vi "Begin.vi"(8 "error in":errorcluster) -> (0 "error out":errorcluster)   [LabVIEW 2019]
doc: "Called before other user functions, this VI is expected to open initial I/O refnums, load in file data, and do all program initialization. Notice that the <B>error out</B> terminal is simply used for data flow. Wiring it to other structures or subVIs ensures that this VI runs first."
uses:
  <vilib>/Rock Robotics/WPI/SafetyOutput/WPI_SafetyOutputConfigMenu.ctl
  <vilib>/Rock Robotics/WPI/DriverStation/WPI_DriverStationRobotMode2.ctl
  <vilib>/Rock Robotics/WPI/Joystick/WPI_JoystickDeviceEnum.ctl
  Robot Global Data.vi
  <vilib>/Rock Robotics/Network Tables/NT Write String Array.vi
  <vilib>/Rock Robotics/WPI/ThirdParty/Phoenix-LabVIEW/Motor Controller/Controls/CTRE_Phoenix_MotorControl_ControlMode.ctl
  <vilib>/Utility/file.llb/Read Delimited Spreadsheet (DBL).vi
  <vilib>/Rock Robotics/WPI/ThirdParty/Phoenix-LabVIEW/Motor Controller/Controls/CTRE_Phoenix_MotorControl_MotionProfileTrajectoryPoint.ctl
  <vilib>/Rock Robotics/WPI/ThirdParty/Phoenix-LabVIEW/Motor Controller/Closed Loop/Motion Profile/CTRE_Phoenix_MotorControl_BufferedTrajectoryPointStream_WriteAll.vi
  <vilib>/Rock Robotics/WPI/ThirdParty/Phoenix-LabVIEW/Motor Controller/Controls/CTRE_Phoenix_MotorControl_FeedbackDevice.ctl
  <vilib>/Rock Robotics/WPI/RobotDrive/WPI_RobotDriveOpen2MotorWithExistingMotors.vi
panel:
  in  "PID":T1
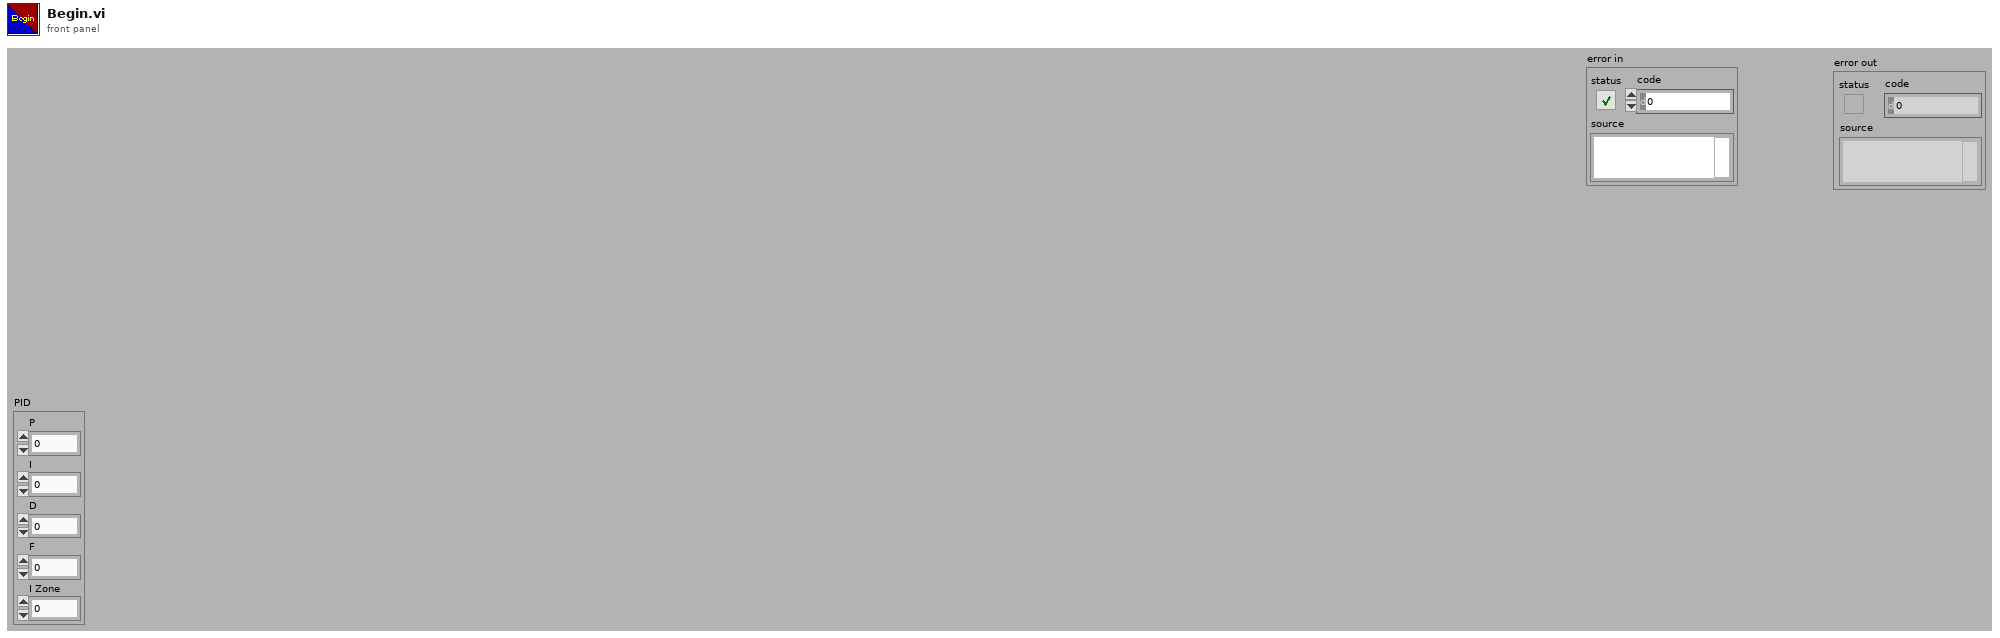
[diagram p1: front panel]
types:
  T1 = cluster{"P":dbl, "I":dbl, "D":dbl, "F":dbl, "I Zone":dbl}
  T2 = enum16{"FollowerType_PercentOutput", "FollowerType_AuxOutput1"}
  T3 = typedef "CTRE_Phoenix_MotorControl_FeedbackDevice.ctl" = i8
  T4 = typedef "CTRE_Phoenix_MotorControl_ControlMode.ctl" = u16
  T5 = typedef "WPI_JoystickDeviceEnum.ctl" = enum16{"USB 0", "USB 1", "USB 2", "USB 3", "USB 4", "USB 5"}
  T6 = typedef "WPI_SafetyOutputConfigMenu.ctl" = enum16{"Enable", "Disable"}
  T7 = typedef "WPI_DriverStationRobotMode2.ctl" = enum16{"Autonomous Disabled", "Autonomous Enabled", "Teleop Disabled", "Teleop Enabled", "Disconnected", "Finish", "Test Disabled", "Test Enabled", "Emergency Stopped"}
  T8 = typedef "WPI_MotorControlDeviceRef.ctl" = cluster{"DeviceStatus":errorcluster, "Type":T9, "PWM":cluster{"PWM Channel":T10, "DeadBand":T11}, "CAN":cluster{"Device Number":u8, "SetOutput VI Ref":variant, "GetOutput VI Ref":variant, "Enable VI Ref":variant, "Disable VI Ref":variant, "Data":variant}, "Invert":bool, "DIO PWM":cluster{"PWM \"Enable\" Channel":T10, "DIOChannel":T12, "PWM Rate":dbl}}
  T9 = typedef "WPI_MotorControlType.ctl" = enum16{"PWM", "CAN", "DIO PWM"}
  T10 = typedef "FPGA_DIOPWMChannel.ctl" = enum8{"PWM 0", "PWM 1", "PWM 2", "PWM 3", "PWM 4", "PWM 5", "PWM 6", "PWM 7", "PWM 8", "PWM 9", "PWM MXP 0", "PWM MXP 1", "PWM MXP 2", "PWM MXP 3", "PWM MXP 4", "PWM MXP 5", "PWM MXP 6", "PWM MXP 7", "PWM MXP 8", "PWM MXP 9", "Invalid"}
  T11 = typedef "WPI_PWMDeadband.ctl" = cluster{"Name":string, "maxPositivePwm":i32, "minPositivePwm":i32, "centerPwm":i32, "maxNegativePwm":i32, "minNegativePwm":i32, "angularRange":u16}
  T12 = typedef "FPGA_DIOChannel.ctl" = enum8{"DIO 0", "DIO 1", "DIO 2", "DIO 3", "DIO 4", "DIO 5", "DIO 6", "DIO 7", "DIO 8", "DIO 9", "DIO MXP 0", "DIO MXP 1", "DIO MXP 2", "DIO MXP 3", "DIO MXP 4", "DIO MXP 5", "DIO MXP 6", "DIO MXP 7", "DIO MXP 8", "DIO MXP 9", "DIO MXP 10", "DIO MXP 11", "DIO MXP 12", "DIO MXP 13", "DIO MXP 14", "DIO MXP 15", "SPI Port CS1", "SPI Port CS2", "SPI Port CS3", "SPI Port MISO", "SPI Port MOSI", "Invalid"}
  T13 = typedef "WPI_RobotDriveDevRef.ctl" = cluster{"DevStatus":errorcluster, "Motors[]":T8[], "Square Inputs":bool, "Max Output":dbl}
  T14 = typedef "WPI_JoystickDevRef.ctl" = cluster{"Device":T5}
  T15 = typedef "CTRE_Phoenix_MotorControl_MotionProfileTrajectoryPoint.ctl" = cluster{"Position":dbl, "Velocity":dbl, "Arbitrary Feed Forward":dbl, "Auxiliary Position":dbl, "Auxiliary Velocity":dbl, "Auxiliary Arbitrary Feed Forward":dbl, "Profile Slot Select":i32, "Auxiliary Profile Slot Select":i32, "isLastPoint?":bool, "Zero Position?":bool, "durationMs":u32, "Use Aux PID?":bool}
  T16 = typedef "CTRE_Phoenix_MotorControl_BufferedTrajectoryPointStream_DeviceRef.ctl" = cluster{"Handle":u64, "Library Path":path}
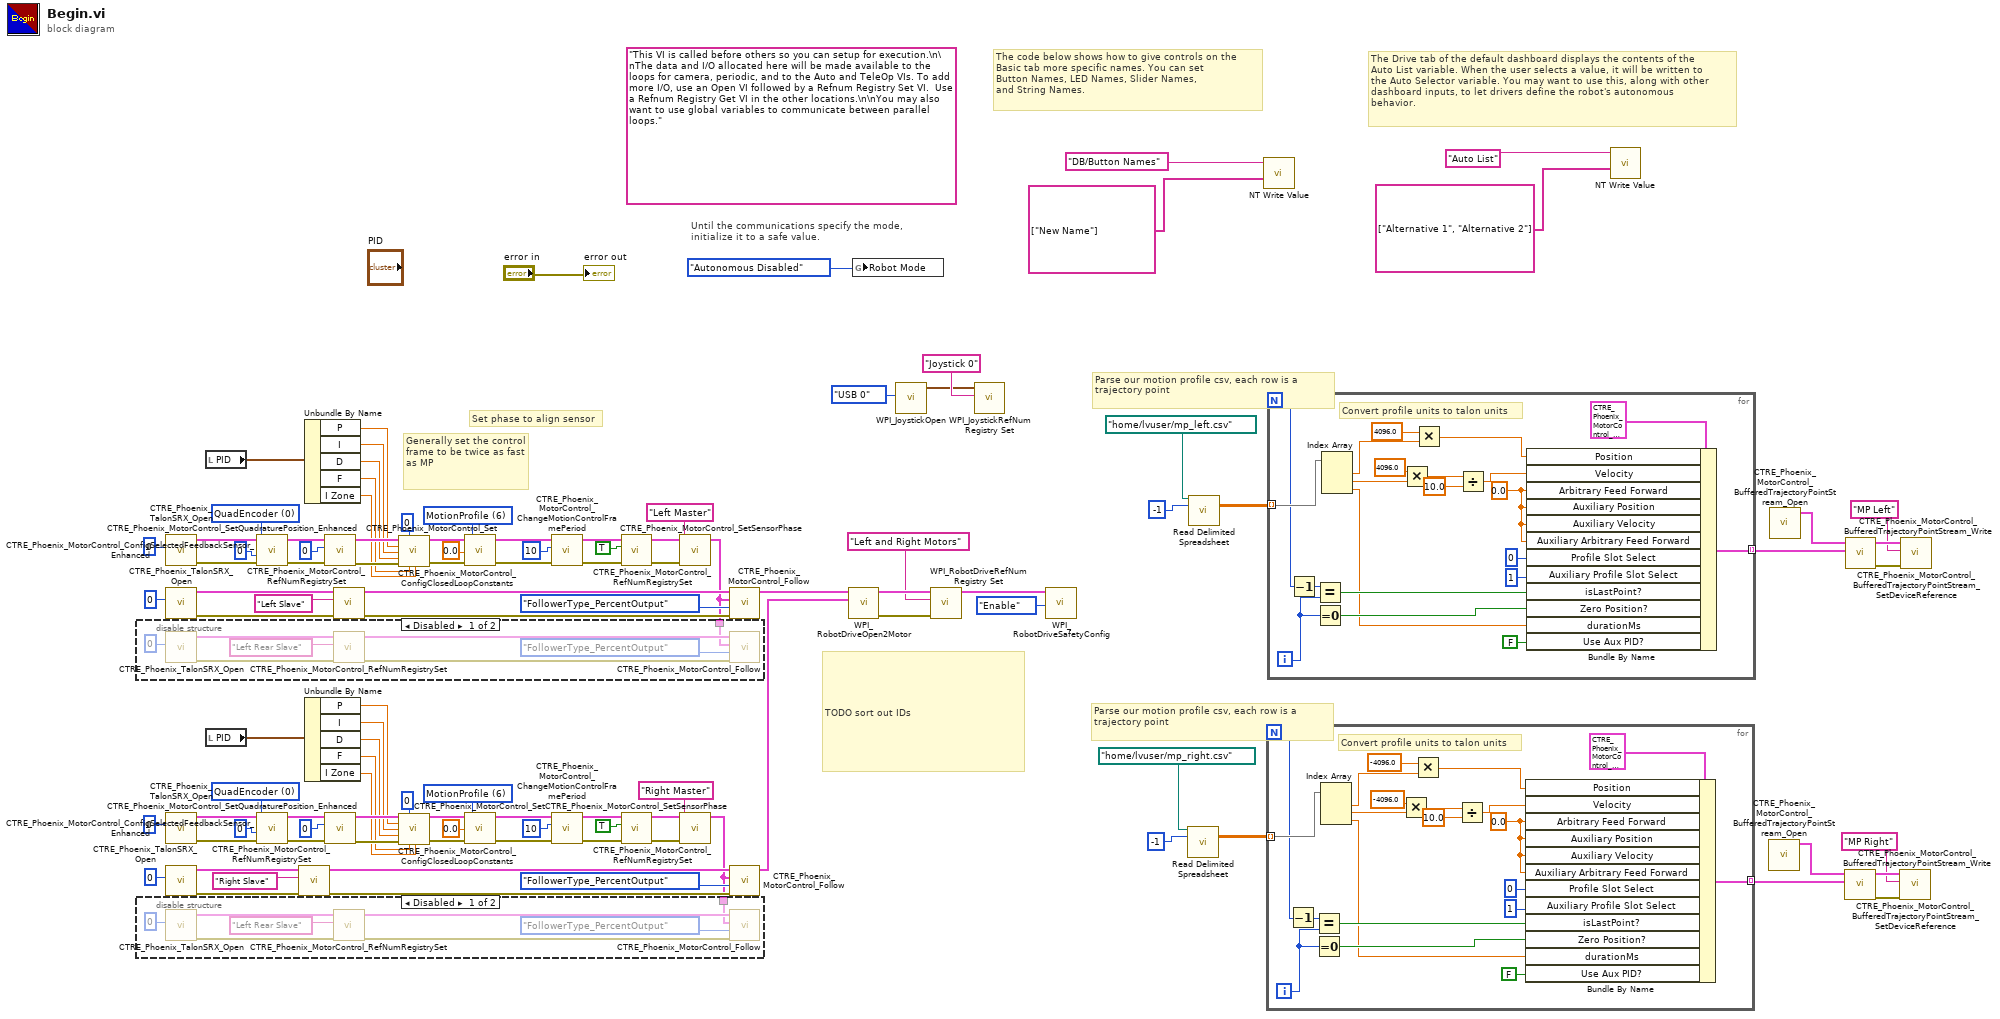
[diagram p0: block diagram]
diagram:
  w40 = T3 0 items=["QuadEncoder"=0, "Analog"=2, "Tachometer"=4, "Pulse Width Encoded Position"=8, "Sensor Sum (S0 + S1)"=9, "Sensor Difference (D0 - D1)"=10, "Remote Source 0"=11, "Remote Source 1"=12, "Software Emulated"=15] ("Feedback Device")
  w48 = T4 6 items=["PercentOutput"=0, "Position"=1, "Velocity"=2, "Current"=3, "Follower"=5, "MotionProfile"=6, "MotionMagic"=7, "MotionMagicArc"=8, "MotionProfileArc"=10, "Disabled"=15] ("Control Mode")
  w77 = T3 0 items=["QuadEncoder"=0, "Analog"=2, "Tachometer"=4, "Pulse Width Encoded Position"=8, "Sensor Sum (S0 + S1)"=9, "Sensor Difference (D0 - D1)"=10, "Remote Source 0"=11, "Remote Source 1"=12, "Software Emulated"=15] ("Feedback Device")
  w93 = T4 6 items=["PercentOutput"=0, "Position"=1, "Velocity"=2, "Current"=3, "Follower"=5, "MotionProfile"=6, "MotionMagic"=7, "MotionMagicArc"=8, "MotionProfileArc"=10, "Disabled"=15] ("Control Mode")
  (unwired) "This VI is called before others so you can setup for execution.\n\nThe data and I/O allocated here will be made available to the loops for camera, periodic, and to the Auto and TeleOp VIs. To add more I/O, use an Open VI followed by a Refnum Registry Set VI.  Use a Refnum Registry Get VI in the other locations.\n\nYou may also want to use global variables to communicate between parallel loops."
  # "Parse our motion profile csv, each row is a trajectory point"
  # "TODO sort out IDs"
  # "Set phase to align sensor"
  # "Generally set the control frame to be twice as fast as MP"
  # "Parse our motion profile csv, each row is a trajectory point"
  # "The Drive tab of the default dashboard displays the contents of the\nAuto List variable. When the user selects a value, it will be written to\nthe Auto Selector variable. You may want to use this, along with other\ndashboard inputs, to let drivers define the robot's autonomous\nbehavior."
  # "The code below shows how to give controls on the\nBasic tab more specific names. You can set\nButton Names, LED Names, Slider Names,\nand String Names."
  # "Until the communications specify the mode,\ninitialize it to a safe value."
  n1 = call <vilib>:"CTRE_Phoenix_TalonSRX_Open.vi"("Device Number"=u8 0) -> ("error out"=w79:errorcluster, "CAN Talon SRX Ref"=w78:T8)  [unwired: 9 in]
  n2 = call <vilib>:"CTRE_Phoenix_TalonSRX_Open.vi"("Device Number"=u8 0) -> ("error out"=w54:errorcluster, "CAN Talon SRX Ref"=w55:T8)  [unwired: 9 in]
  n3 = call <vilib>:"CTRE_Phoenix_TalonSRX_Open.vi"("Device Number"=u8 0) -> ("error out"=w42:errorcluster, "CAN Talon SRX Ref"=w41:T8)  [unwired: 9 in]
  n4 = call <vilib>:"CTRE_Phoenix_TalonSRX_Open.vi"("Device Number"=u8 0) -> ("error out"=w17:errorcluster, "CAN Talon SRX Ref"=w18:T8)  [unwired: 9 in]
  n5 = local read "PID"() -> (w60:T1)
  n6 = local read "PID"() -> (w23:T1)
  n7 = call <vilib>:"CTRE_Phoenix_MotorControl_ConfigSelectedFeedbackSensor_Enhanced.vi"("error in (no error)"=w79, "pidLoopIdx"=0, "Feedback Device"=w77, "PhoenixMotorControlDevRef"=w78) -> ("error out"=w74:errorcluster, "PhoenixMotorControlDevRef"=w75:T8)  [unwired: 6 in]
  n8 = call <vilib>:"CTRE_Phoenix_MotorControl_ConfigSelectedFeedbackSensor_Enhanced.vi"("error in (no error)"=w42, "pidLoopIdx"=0, "Feedback Device"=w40, "PhoenixMotorControlDevRef"=w41) -> ("error out"=w37:errorcluster, "PhoenixMotorControlDevRef"=w38:T8)  [unwired: 6 in]
  n9 = call <vilib>:"CTRE_Phoenix_MotorControl_RefNumRegistrySet.vi"("error in (no error)"=w17, "refnum name"="Right Slave", "PhoenixMotorControlDevRef"=w18) -> ("error out"=w13:errorcluster, "PhoenixMotorControlDevRef"=w15:T8)  [unwired: 7 in]
  n10 = Unbundle By Name(w60) -> ("P"=w70:dbl, "I"=w69:dbl, "D"=w68:dbl, "F"=w67:dbl, "I Zone"=w66:dbl)
  n11 = Unbundle By Name(w23) -> ("P"=w33:dbl, "I"=w32:dbl, "D"=w31:dbl, "F"=w30:dbl, "I Zone"=w29:dbl)
  n12 = call <vilib>:"CTRE_Phoenix_MotorControl_SetQuadraturePosition_Enhanced.vi"("error in (no error)"=w74, "New Position"=0, "PhoenixMotorControlDevRef"=w75) -> ("error out"=w71:errorcluster, "PhoenixMotorControlDevRef"=w72:T8)  [unwired: 7 in]
  n13 = call <vilib>:"CTRE_Phoenix_MotorControl_SetQuadraturePosition_Enhanced.vi"("error in (no error)"=w37, "New Position"=0, "PhoenixMotorControlDevRef"=w38) -> ("error out"=w34:errorcluster, "PhoenixMotorControlDevRef"=w35:T8)  [unwired: 7 in]
  n14 = call <vilib>:"CTRE_Phoenix_MotorControl_RefNumRegistrySet.vi"("error in (no error)"=w54, "refnum name"="Left Slave", "PhoenixMotorControlDevRef"=w55) -> ("error out"=w50:errorcluster, "PhoenixMotorControlDevRef"=w52:T8)  [unwired: 7 in]
  n15 = call <vilib>:"CTRE_Phoenix_MotorControl_ConfigClosedLoopConstants.vi"("PhoenixMotorControlDevRef"=w72, "slotIdx"=0, "P"=w70, "I"=w69, "D"=w68, "error in (no error)"=w71, "F"=w67, "I Zone"=w66) -> ("PhoenixMotorControlDevRef"=w64:T8, "error out"=w63:errorcluster)  [unwired: 6 in]
  n16 = call <vilib>:"CTRE_Phoenix_MotorControl_ConfigClosedLoopConstants.vi"("PhoenixMotorControlDevRef"=w35, "slotIdx"=0, "P"=w33, "I"=w32, "D"=w31, "error in (no error)"=w34, "F"=w30, "I Zone"=w29) -> ("PhoenixMotorControlDevRef"=w27:T8, "error out"=w26:errorcluster)  [unwired: 6 in]
  n17 = call <vilib>:"CTRE_Phoenix_MotorControl_Set.vi"("error in (no error)"=w63, "Output"=0.0, "Control Mode"=w93, "PhoenixMotorControlDevRef"=w64) -> ("error out"=w62:errorcluster, "PhoenixMotorControlDevRef"=w82:T8)  [unwired: 6 in]
  n18 = call <vilib>:"CTRE_Phoenix_MotorControl_Set.vi"("error in (no error)"=w26, "Output"=0.0, "Control Mode"=w48, "PhoenixMotorControlDevRef"=w27) -> ("error out"=w25:errorcluster, "PhoenixMotorControlDevRef"=w45:T8)  [unwired: 6 in]
  n19 = call <vilib>:"CTRE_Phoenix_MotorControl_ChangeMotionControlFramePeriod.vi"("error in"=w62, "periodMs"=10, "PhoenixMotorControlDevRef"=w82) -> ("error out"=w61:errorcluster, "PhoenixMotorControlDevRef"=w80:T8)  [unwired: 7 in]
  n20 = call <vilib>:"CTRE_Phoenix_MotorControl_ChangeMotionControlFramePeriod.vi"("error in"=w25, "periodMs"=10, "PhoenixMotorControlDevRef"=w45) -> ("error out"=w24:errorcluster, "PhoenixMotorControlDevRef"=w43:T8)  [unwired: 7 in]
  n21 = call <vilib>:"CTRE_Phoenix_MotorControl_SetSensorPhase.vi"("error in (no error)"=w61, "PhaseSensor"=TRUE, "PhoenixMotorControlDevRef"=w80) -> ("error out"=w59:errorcluster, "PhoenixMotorControlDevRef"=w58:T8)  [unwired: 7 in]
  n22 = call <vilib>:"CTRE_Phoenix_MotorControl_SetSensorPhase.vi"("error in (no error)"=w24, "PhaseSensor"=TRUE, "PhoenixMotorControlDevRef"=w43) -> ("error out"=w22:errorcluster, "PhoenixMotorControlDevRef"=w21:T8)  [unwired: 7 in]
  n23 = call <vilib>:"CTRE_Phoenix_MotorControl_RefNumRegistrySet.vi"("error in (no error)"=w59, "refnum name"="Left Master", "PhoenixMotorControlDevRef"=w58) -> ("PhoenixMotorControlDevRef"=w2:T8)  [unwired: 7 in, 1 out]
  n24 = disable-structure shown="Disabled" {
    disable-tunnel: w2 -> [w109 _]
    frame Disabled {
      n25 = call <vilib>:"CTRE_Phoenix_TalonSRX_Open.vi"("Device Number"=u8 0) -> ("error out"=w114:errorcluster, "CAN Talon SRX Ref"=w115:T8)  [unwired: 9 in]
      n26 = call <vilib>:"CTRE_Phoenix_MotorControl_RefNumRegistrySet.vi"("error in (no error)"=w114, "refnum name"="Left Rear Slave", "PhoenixMotorControlDevRef"=w115) -> ("error out"=w110:errorcluster, "PhoenixMotorControlDevRef"=w112:T8)  [unwired: 7 in]
      n27 = call <vilib>:"CTRE_Phoenix_MotorControl_Follow.vi"("error in (no error)"=w110, "FollowerType"=T2."FollowerType_PercentOutput", "Master Controller to Follow"=w109, "PhoenixMotorControlDevRef"=w112) -> ()  [unwired: 6 in, 2 out]
    }
    frame Enabled {
    }
  }
  n28 = call <vilib>:"CTRE_Phoenix_MotorControl_RefNumRegistrySet.vi"("error in (no error)"=w22, "refnum name"="Right Master", "PhoenixMotorControlDevRef"=w21) -> ("PhoenixMotorControlDevRef"=w1:T8)  [unwired: 7 in, 1 out]
  n29 = disable-structure shown="Disabled" {
    disable-tunnel: w1 -> [w117 _]
    frame Disabled {
      n30 = call <vilib>:"CTRE_Phoenix_TalonSRX_Open.vi"("Device Number"=u8 0) -> ("error out"=w122:errorcluster, "CAN Talon SRX Ref"=w123:T8)  [unwired: 9 in]
      n31 = call <vilib>:"CTRE_Phoenix_MotorControl_RefNumRegistrySet.vi"("error in (no error)"=w122, "refnum name"="Left Rear Slave", "PhoenixMotorControlDevRef"=w123) -> ("error out"=w118:errorcluster, "PhoenixMotorControlDevRef"=w120:T8)  [unwired: 7 in]
      n32 = call <vilib>:"CTRE_Phoenix_MotorControl_Follow.vi"("error in (no error)"=w118, "FollowerType"=T2."FollowerType_PercentOutput", "Master Controller to Follow"=w117, "PhoenixMotorControlDevRef"=w120) -> ()  [unwired: 6 in, 2 out]
    }
    frame Enabled {
    }
  }
  n33 = call <vilib>:"CTRE_Phoenix_MotorControl_Follow.vi"("error in (no error)"=w50, "FollowerType"=T2."FollowerType_PercentOutput", "Master Controller to Follow"=w2, "PhoenixMotorControlDevRef"=w52) -> ("PhoenixMotorControlDevRef"=w12:T8)  [unwired: 6 in, 1 out]
  n34 = call <vilib>:"CTRE_Phoenix_MotorControl_Follow.vi"("error in (no error)"=w13, "FollowerType"=T2."FollowerType_PercentOutput", "Master Controller to Follow"=w1, "PhoenixMotorControlDevRef"=w15) -> ("PhoenixMotorControlDevRef"=w11:T8)  [unwired: 6 in, 1 out]
  n35 = call-poly <vilib>:"WPI_RobotDriveOpen2Motor.vi"("Right Motor Dev Ref"=w11, "Left Motor Dev Ref"=w12) -> ("error out"=w100:errorcluster, "RobotDriveDevRef"=w102:T13)  [unwired: 3 in, 5 out]
  n36 = global write "Robot Global Data.vi" "Robot Mode"(WPI_DriverStationRobotMode2."Autonomous Disabled" ("Robot Mode")) -> ()
  n37 = call <vilib>:"WPI_JoystickOpen.vi"("JoystickDevice"=WPI_JoystickDeviceEnum."USB 0") -> ("JoystickDevRef"=w96:T14)  [unwired: 10 in]
  n38 = call <vilib>:"WPI_RobotDriveRefNum Registry Set.vi"("error in (no error)"=w100, "refnum name"="Left and Right Motors", "RobotDriveDevRef"=w102) -> ("RobotDriveDevRef"=w99:T13)  [unwired: 1 in, 7 out]
  n39 = call <vilib>:"WPI_JoystickRefNum Registry Set.vi"("refnum name"="Joystick 0", "JoystickDevRef"=w96) -> ()  [unwired: 8 in, 2 out]
  n40 = call <vilib>:"WPI_RobotDriveSafetyConfig.vi"("mode"=WPI_SafetyOutputConfigMenu."Enable", "RobotDriveDevRef"=w99) -> ()  [unwired: 8 in, 2 out]
  n41 = call-poly <vilib>:"Read Delimited Spreadsheet.vi"("file path (dialog if empty)"=path "/home/lvuser/mp_right.csv" ("file path (use dialog)"), "number of rows (all:-1)"=-1) -> ("all rows"=w8:dbl[][])  [unwired: 8 in, 5 out]
  n42 = call-poly <vilib>:"Read Delimited Spreadsheet.vi"("file path (dialog if empty)"=path "/home/lvuser/mp_left.csv" ("file path (use dialog)"), "number of rows (all:-1)"=-1) -> ("all rows"=w89:dbl[][])  [unwired: 8 in, 5 out]
  n43 = call-poly <vilib>:"NT Write Value.vi"("String Array"=string[] ["New Name"], "Name"="DB/Button Names") -> ()  [unwired: 9 in, 1 out]
  n44 = for {
    N -> [w138]
    tunnel: w8 -> [w144] mode=indexing
    tunnel: [w134] -> w7 mode=indexing
    i -> [w137]
    w143 = 0.0 ("Arbitrary Feed Forward")
    # "Convert profile units to talon units"
    n45 = Decrement(x=w138) -> (x-1=w139:i32)
    n46 = Equal?(x=w139, y=w137) -> (x = y?=w140:bool)
    n47 = Equal To 0?(x=w137) -> (x = 0?=w136:bool)
    n48 = Index Array(array=w144) -> (element #1=w132:dbl, element #2=w126:dbl, element #3=w133:dbl)  [unwired: 3 in]
    n49 = Multiply(x=-4096.0, y=w126) -> (x*y=w128:dbl)
    n50 = Multiply(x=-4096.0, y=w132) -> (x*y=w130:dbl)
    n51 = Divide(x=w128, y=10.0) -> (x/y=w125:dbl)
    n52 = Bundle By Name(cluster=T15 {"Position"=0.0, "Velocity"=0.0, "Arbitrary Feed Forward"=0.0, "Auxiliary Position"=0.0, "Auxiliary Velocity"=0.0, "Auxiliary Arbitrary Feed Forward"=0.0, "Profile Slot Select"=0, "Auxiliary Profile Slot Select"=0, "isLastPoint?"=FALSE, "Zero Position?"=FALSE, "durationMs"=0, "Use Aux PID?"=FALSE} ("Trajectory Point"), "Position"=w130, "Velocity"=w125, "Arbitrary Feed Forward"=w143, "Auxiliary Position"=w143, "Auxiliary Velocity"=w143, "Auxiliary Arbitrary Feed Forward"=w143, "Profile Slot Select"=0, "Auxiliary Profile Slot Select"=1, "isLastPoint?"=w140, "Zero Position?"=w136, "durationMs"=w133, "Use Aux PID?"=FALSE) -> (w134:T15)
  }
  n53 = for {
    N -> [w159]
    tunnel: w89 -> [w165] mode=indexing
    tunnel: [w155] -> w88 mode=indexing
    i -> [w158]
    w164 = 0.0 ("Arbitrary Feed Forward")
    # "Convert profile units to talon units"
    n54 = Decrement(x=w159) -> (x-1=w160:i32)
    n55 = Equal?(x=w160, y=w158) -> (x = y?=w161:bool)
    n56 = Equal To 0?(x=w158) -> (x = 0?=w157:bool)
    n57 = Index Array(array=w165) -> (element #1=w153:dbl, element #2=w147:dbl, element #3=w154:dbl)  [unwired: 3 in]
    n58 = Multiply(x=4096.0, y=w147) -> (x*y=w149:dbl)
    n59 = Multiply(x=4096.0, y=w153) -> (x*y=w151:dbl)
    n60 = Divide(x=w149, y=10.0) -> (x/y=w146:dbl)
    n61 = Bundle By Name(cluster=T15 {"Position"=0.0, "Velocity"=0.0, "Arbitrary Feed Forward"=0.0, "Auxiliary Position"=0.0, "Auxiliary Velocity"=0.0, "Auxiliary Arbitrary Feed Forward"=0.0, "Profile Slot Select"=0, "Auxiliary Profile Slot Select"=0, "isLastPoint?"=FALSE, "Zero Position?"=FALSE, "durationMs"=0, "Use Aux PID?"=FALSE} ("Trajectory Point"), "Position"=w151, "Velocity"=w146, "Arbitrary Feed Forward"=w164, "Auxiliary Position"=w164, "Auxiliary Velocity"=w164, "Auxiliary Arbitrary Feed Forward"=w164, "Profile Slot Select"=0, "Auxiliary Profile Slot Select"=1, "isLastPoint?"=w161, "Zero Position?"=w157, "durationMs"=w154, "Use Aux PID?"=FALSE) -> (w155:T15)
  }
  n62 = call-poly <vilib>:"NT Write Value.vi"("String Array"=string[] ["Alternative 1", "Alternative 2"], "Name"="Auto List") -> ()  [unwired: 9 in, 1 out]
  n63 = call <vilib>:"CTRE_Phoenix_MotorControl_BufferedTrajectoryPointStream_Open.vi"() -> ("BufferedTrajectoryPointStream_DevRef"=w6:T16)  [unwired: 10 in, 1 out]
  n64 = call <vilib>:"CTRE_Phoenix_MotorControl_BufferedTrajectoryPointStream_Open.vi"() -> ("BufferedTrajectoryPointStream_DevRef"=w87:T16)  [unwired: 10 in, 1 out]
  n65 = call-poly <vilib>:"CTRE_Phoenix_MotorControl_BufferedTrajectoryPointStream_Write.vi"("Motion Profile Trajectory Point Array"=w7, "BufferedTrajectoryPointStream_DevRef"=w6) -> ("error out"=w4:errorcluster, "BufferedTrajectoryPointStream_DevRef"=w5:T16)  [unwired: 8 in]
  n66 = call-poly <vilib>:"CTRE_Phoenix_MotorControl_BufferedTrajectoryPointStream_Write.vi"("Motion Profile Trajectory Point Array"=w88, "BufferedTrajectoryPointStream_DevRef"=w87) -> ("error out"=w85:errorcluster, "BufferedTrajectoryPointStream_DevRef"=w86:T16)  [unwired: 8 in]
  n67 = call <vilib>:"CTRE_Phoenix_MotorControl_BufferedTrajectoryPointStream_SetDeviceReference.vi"("error in (no error)"=w4, "refnum name"="MP Right", "BufferedTrajectoryPointStream_DevRef"=w5) -> ()  [unwired: 7 in, 2 out]
  n68 = call <vilib>:"CTRE_Phoenix_MotorControl_BufferedTrajectoryPointStream_SetDeviceReference.vi"("error in (no error)"=w85, "refnum name"="MP Left", "BufferedTrajectoryPointStream_DevRef"=w86) -> ()  [unwired: 7 in, 2 out]
  "error out" <- "error in"
